vi "Read TEC.vi"(8 "error in (no error)":errorcluster, 11 "TEC Controller in":refnum<class "TEC Controller.lvclass">) -> (0 "error out":errorcluster, 2 "TEC":refnum<vi>, 3 "TEC Controller out":refnum<class "TEC Controller.lvclass">)   [LabVIEW 2014, in "Humidifier Test Lib.lvlib" / "TEC Controller.lvclass"]
uses:
  TEC Controller.lvclass
  TEC Controller.lvclass/TEC Controller.ctl
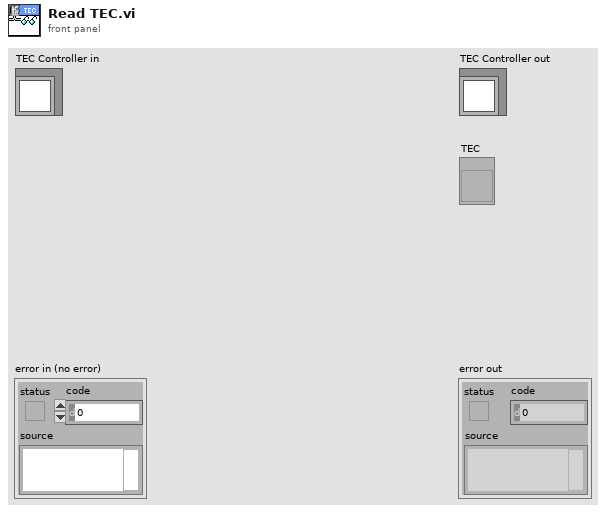
[diagram p1: front panel]
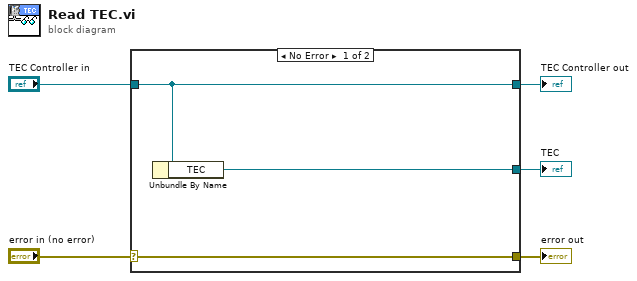
[diagram p0: block diagram]
diagram:
  n1 = case shown="No Error" "error in (no error)" {
    selector: "error in (no error)" -> [w8 w9]
    tunnel: [w8 w9] -> w4
    tunnel: [w7 w10] -> w2
    tunnel: "TEC Controller in" -> [w7 w10]
    tunnel: [w6 _] -> w1
    frame No Error {
      n2 = Unbundle By Name(w7) -> ("TEC"=w6:refnum<vi>)
    }
    frame Error {
    }
  }
  "error out" <- w4
  "TEC Controller out" <- w2
  "TEC" <- w1
